vi "Parse Tag Key.vi"(8 "Error In":errorcluster, 11 "Parser In":refnum<class "Parser.lvclass">) -> (0 "Error Out":errorcluster, 3 "Parser Out":refnum<class "Parser.lvclass">)   [LabVIEW 2018, in "Toolkit.lvlib" / "Parser.lvclass"]
uses:
  Parser.lvclass
  Parser.lvclass/Parser.ctl
  API/Controls/States.ctl
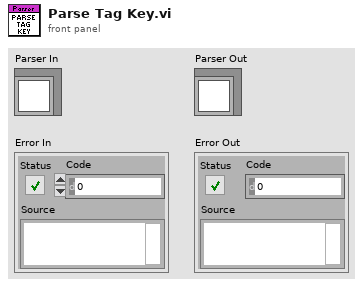
[diagram p1: front panel]
types:
  T1 = typedef "Toolkit.lvlib/Parser.lvclass/States.ctl" = enum16{"Text", "Open Delimiter", "Tag Type", "Tag Key", "Close Delimiter"}
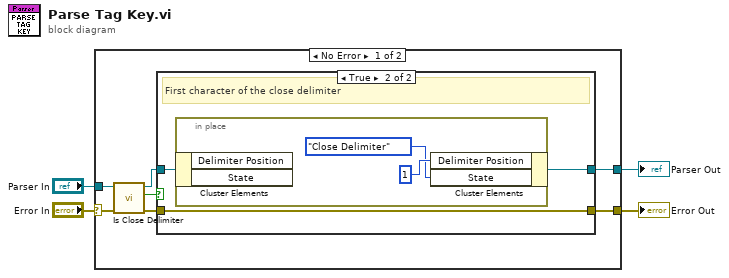
[diagram p0: block diagram]
diagram:
  n1 = case shown="No Error" "Error In" {
    selector: "Error In" -> [w11 w20]
    tunnel: "Parser In" -> [w10 w19]
    tunnel: [w6 w19] -> w3
    tunnel: [w5 w20] -> w1
    frame No Error {
      n2 = call "Is Close Delimiter.vi"("Error In"=w11, "Parser In"=w10) -> ("Error Out"=w7:errorcluster, "Close Delimiter"=w9:bool, "Parser Out"=w8:refnum<class "Parser.lvclass">)  [unwired: 7 in]
      n3 = case shown="True" w9 {
        tunnel: w8 -> [w12 w15]
        tunnel: w7 -> [w13 w16]
        tunnel: [w12 w14] -> w6
        tunnel: [w13 w16] -> w5
        frame False {
          # "Character is just text"
        }
        frame True {
          # "First character of the close delimiter"
          n4 = in-place {
            n5 = in-place-cluster #1(w15) -> ()  [unwired: 2 out]
            n6 = in-place-cluster #1("Delimiter Position"=1, "State"=States."Close Delimiter") -> (w14:refnum<class "Parser.lvclass">)
          }
        }
      }
    }
    frame Error {
    }
  }
  "Parser Out" <- w3
  "Error Out" <- w1
